vi "Global 5.vi"() -> ()   [LabVIEW 2017]
panel:
  out "Boolean":bool
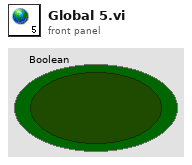
[diagram p1: front panel]
diagram:
